vi "ChildModule.Dock Pane.vi"(8 "error in (no error)":errorcluster, 10 "Sub Panel":refnum<vi>, 11 "Module Name":string) -> (0 "error out":errorcluster)   [LabVIEW 2016]
uses:
  <vilib>/KATE/Module/Public/Action - Window Tasks.ctl
  <vilib>/KATE/Module/Module Utils.lvlib
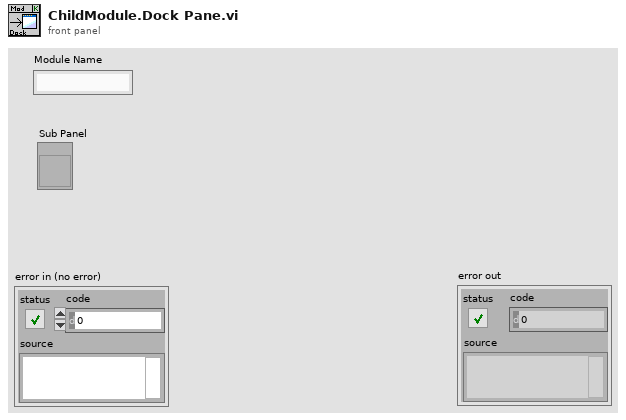
[diagram p1: front panel]
types:
  T1 = typedef "KATE_Lib.lvlib/Module Utils.lvlib/Action - Window Tasks.ctl" = enum16{"Resize()", "Show Panel(Bool)", "Show Scroll Bars(Bool)", "Dock to SubPanel(SubPanel Ref)", "Undock from SubPanel()", "Return to SubPanel()", "Go To Maint Tab()", "Show Maint Tab(Bool)", "Open Block Diagram()"}
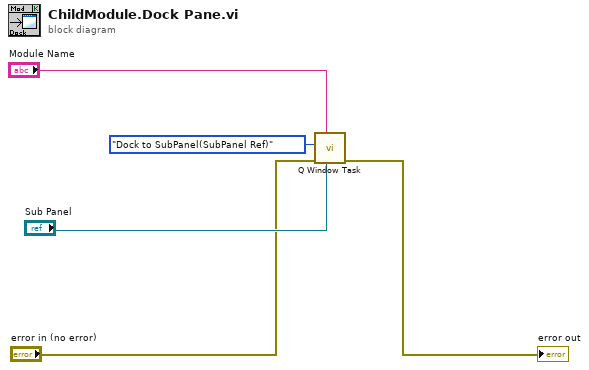
[diagram p0: block diagram]
diagram:
  n1 = call <vilib>:"Q Window Task.vi"("Sub Panel"="Sub Panel", "Q Name"="Module Name", "error in"="error in (no error)", "Action"=Action_-_Window_Tasks."Dock to SubPanel(SubPanel Ref)") -> ("error out"=→"error out":errorcluster)  [unwired: 6 in, 1 out]
